vi "ProbeAdjustment.vi"() -> ()   [LabVIEW 2014]
uses:
  <vilib>/rvi/Emulation/niFpgaSctlEmulationGetInTimedLoop.vi
  <vilib>/rvi/Emulation/niFpgaProcessEmulError.vi
  <vilib>/rvi/eio/common/nirviEmuTemplateMethod_errors.vi
  <vilib>/rvi/Emulation/niFpgaGetClockAttributes.vi
  <vilib>/rvi/Emulation/niFpgaEmulationReportErrorSimple.vi
  <vilib>/rvi/Emulation/niFpgaCriticalErrorInLSC.vi
  <vilib>/eio/EIONode/EIONode.xnode
panel:
  out "NewRefCurrIndex":i16
  out "preCurrIndex":i16
  out "Reversing?":bool=TRUE
  in  "Terminal":bool=TRUE
  out "InPlace?":bool
  out "Approached?":bool
  in  "stop":bool
  out "PIZPos":i16
  in  "ProbeBrokenIndex":i16
  in  "ScanNumToRefresh":i16
  in  "ThresholdIndex":i16
  in  "stepMultiplier/0.305nm":i16
  in  "refCurrIndex":i16
  in  "Sleep ms":i16
  in  "ThresholdLowerBound":i16
  in  "ThresholdUpperBound":i16
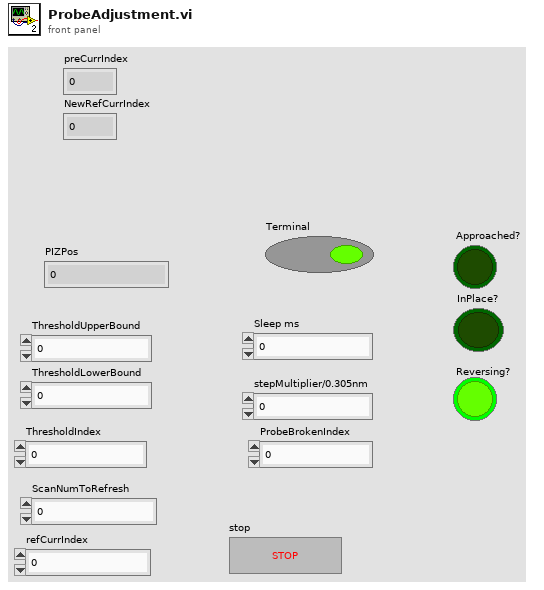
[diagram p1: front panel]
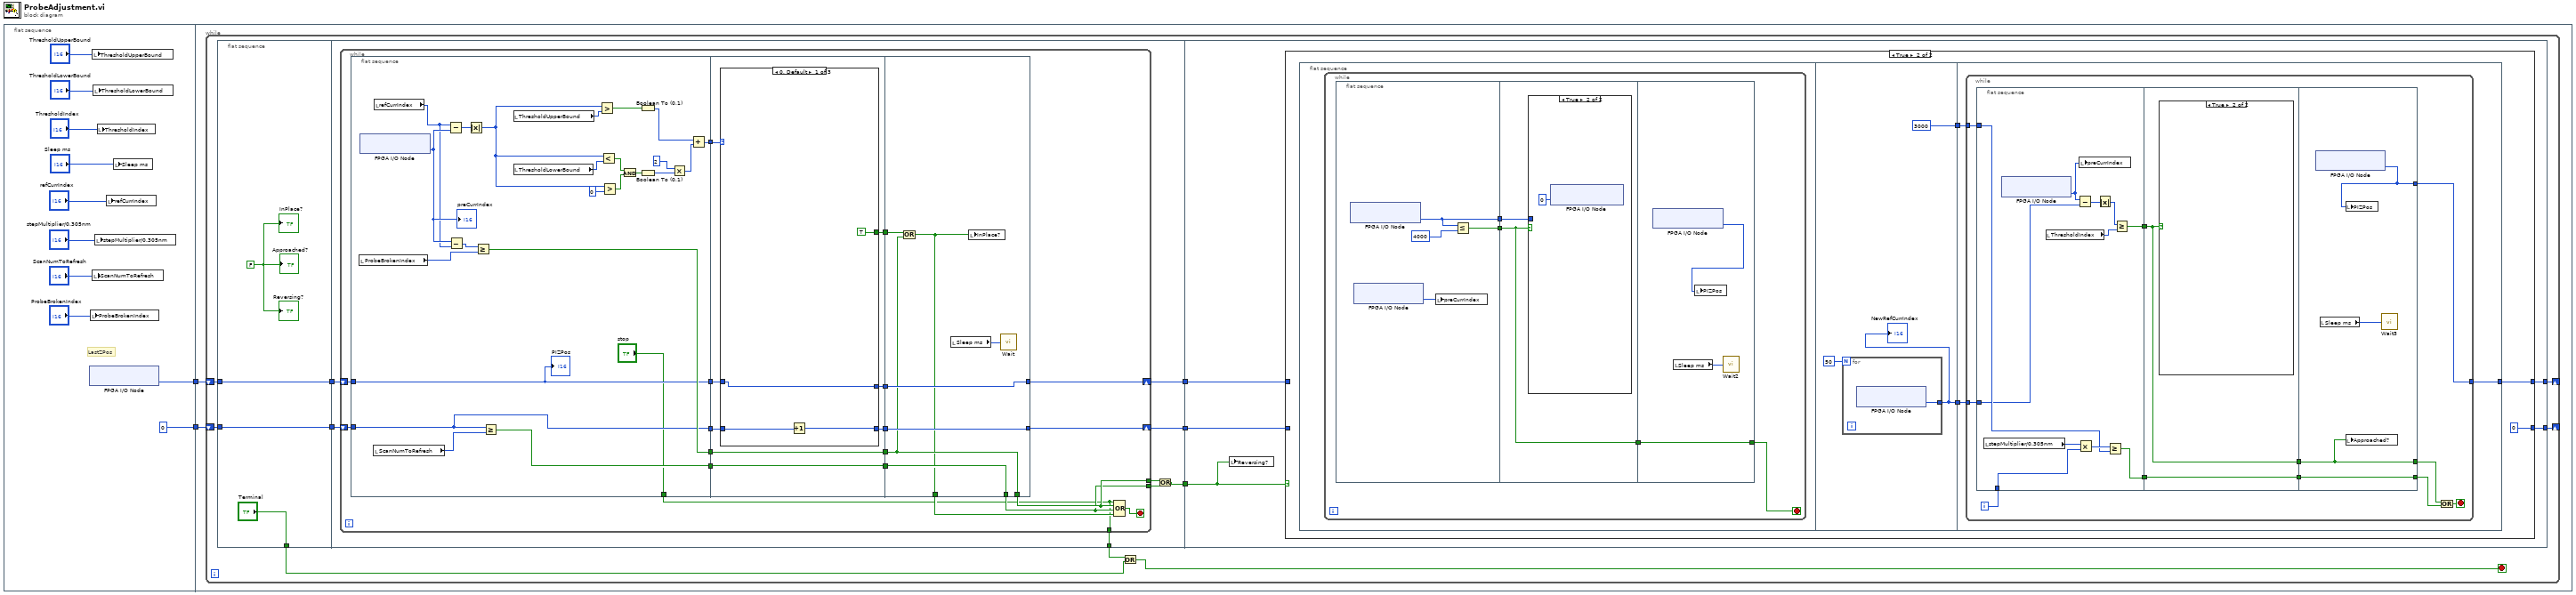
[diagram p0: block diagram]
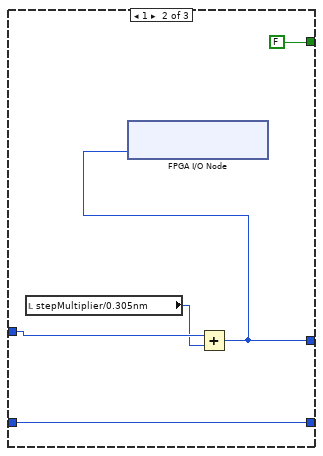
[diagram p2: hidden frame]
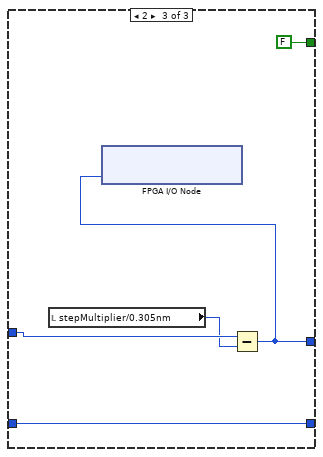
[diagram p3: hidden frame]
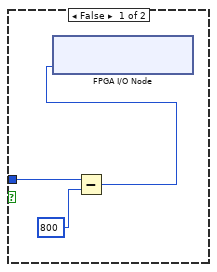
[diagram p5: hidden frame]
diagram:
  n1 = flat-sequence {
    tunnel: [w4] -> w2
    tunnel: [i16 0] -> w1
    tunnel: w2 -> [w13]
    tunnel: w1 -> [w14]
    frame #0 {
      # "LastZPos"
      n2 = xnode "FPGA I/O Node"() -> ("Connector0/AI0"=w4:i16)  [unwired: 1 in, 1 out]
      n3 = local write "ProbeBrokenIndex"("ProbeBrokenIndex") -> ()
      n4 = local write "ThresholdUpperBound"("ThresholdUpperBound") -> ()
      n5 = local write "ScanNumToRefresh"("ScanNumToRefresh") -> ()
      n6 = local write "ThresholdLowerBound"("ThresholdLowerBound") -> ()
      n7 = local write "stepMultiplier/0.305nm"("stepMultiplier/0.305nm") -> ()
      n8 = local write "ThresholdIndex"("ThresholdIndex") -> ()
      n9 = local write "refCurrIndex"("refCurrIndex") -> ()
      n10 = local write "Sleep ms"("Sleep ms") -> ()
    }
    frame #1 {
      n11 = while {
        shift-right: [w22] -> _
        shift-left: w14 -> [w26]
        shift-right: [w20] -> _
        shift-left: w13 -> [w25]
        stop <- w15 stop-if-true
        n12 = flat-sequence {
          tunnel: w25 -> [w29]
          tunnel: w26 -> [w30]
          tunnel: [w30] -> w24
          tunnel: [w29] -> w23
          tunnel: ["Terminal"] -> w16
          tunnel: [w36] -> w17
          tunnel: w24 -> [w38]
          tunnel: w23 -> [w37]
          tunnel: [w35] -> w21
          tunnel: [w34] -> w19
          tunnel: [w31] -> w18
          tunnel: w21 -> [w114]
          tunnel: w19 -> [w112]
          tunnel: [w115] -> w22
          tunnel: [w113] -> w20
          tunnel: w18 -> [w111]
          frame #0 {
            w27 = FALSE
            "Approached?" <- w27
            "InPlace?" <- w27
            "Reversing?" <- w27
          }
          frame #1 {
            n13 = while {
              shift-right: [w46] -> w34
              shift-left: w37 -> [w52]
              shift-right: [w48] -> w35
              shift-left: w38 -> [w53]
              tunnel: [w39] -> w36
              tunnel: [w41] -> w33
              tunnel: [w40] -> w32
              stop <- w43 stop-if-true
              n14 = flat-sequence {
                tunnel: [w66] -> w57
                tunnel: [w63] -> w54
                tunnel: w53 -> [w59]
                tunnel: w52 -> [w62]
                tunnel: [w62] -> w51
                tunnel: [w59] -> w50
                tunnel: [w60] -> w45
                tunnel: ["stop"] -> w39
                tunnel: w57 -> [w89]
                tunnel: [w88] -> w56
                tunnel: [w87] -> w55
                tunnel: w54 -> [w87]
                tunnel: w51 -> [w86]
                tunnel: w50 -> [w83]
                tunnel: [w84] -> w49
                tunnel: [w85] -> w47
                tunnel: w45 -> [w82]
                tunnel: [w82] -> w44
                tunnel: w56 -> [w109]
                tunnel: w55 -> [w106]
                tunnel: w49 -> [w107]
                tunnel: [w107] -> w48
                tunnel: [w108] -> w46
                tunnel: w47 -> [w108]
                tunnel: [w106] -> w41
                tunnel: [w105] -> w40
                tunnel: w44 -> [w105]
                tunnel: [w104] -> w42
                frame #0 {
                  n15 = local read "ProbeBrokenIndex"() -> (w64:i16)
                  n16 = xnode "FPGA I/O Node"() -> ("Connector0/AI1"=w78:i16)  [unwired: 1 in, 1 out]
                  "preCurrIndex" <- w78
                  n17 = local read "ScanNumToRefresh"() -> (w61:i16)
                  n18 = local read "refCurrIndex"() -> (w77:i16)
                  n19 = Subtract(x=w77, y=w78) -> (x-y=w79:i16)
                  n20 = Subtract(x=w78, y=w77) -> (x-y=w65:i16)
                  n21 = Absolute Value(x=w79) -> (abs(x)=w76:i16)
                  n22 = Greater Or Equal?(x=w65, y=w64) -> (x >= y?=w63:bool)
                  n23 = Greater Or Equal?(x=w59, y=w61) -> (x >= y?=w60:bool)
                  n24 = local read "ThresholdUpperBound"() -> (w81:i16)
                  n25 = local read "ThresholdLowerBound"() -> (w80:i16)
                  n26 = Greater?(x=w76, y=w81) -> (0:w69:bool)
                  n27 = Less?(x=w76, y=w80) -> (x < y?=w74:bool)
                  n28 = Greater?(x=w76, y=i16 0) -> (0:w73:bool)
                  n29 = And(x=w74, y=w73) -> (x .and. y?=w72:bool)
                  n30 = Boolean To (0,1)(Boolean=w69) -> (0, 1=w67:i16)
                  n31 = Boolean To (0,1)(Boolean=w72) -> (0, 1=w71:i16)
                  n32 = Multiply(x=i16 2, y=w71) -> (x*y=w68:i16)
                  n33 = Add(x=w67, y=w68) -> (x+y=w66:i16)
                  "PIZPos" <- w62
                }
                frame #1 {
                  n34 = case shown="0, Default" w89 {
                    tunnel: [TRUE FALSE FALSE] -> w88
                    tunnel: w86 -> [w92 w97 w102]
                    tunnel: [w92 w94 w99] -> w85
                    tunnel: [w90 w95 w100] -> w84
                    tunnel: w83 -> [w91 w95 w100]
                    frame 0, Default {
                      n35 = Increment(x=w91) -> (x+1=w90:i16)
                    }
                    frame 1 {
                      n36 = local read "stepMultiplier/0.305nm"() -> (w96:i16)
                      n37 = Add(x=w97, y=w96) -> (x+y=w94:i16)
                      n38 = xnode "FPGA I/O Node"("Connector0/AO0"=w94) -> ()  [unwired: 1 in, 1 out]
                    }
                    frame 2 {
                      n39 = local read "stepMultiplier/0.305nm"() -> (w101:i16)
                      n40 = Subtract(x=w102, y=w101) -> (x-y=w99:i16)
                      n41 = xnode "FPGA I/O Node"("Connector0/AO0"=w99) -> ()  [unwired: 1 in, 1 out]
                    }
                  }
                }
                frame #2 {
                  n42 = Compound Arithmetic op=OR(w109, w106) -> (w104:bool)
                  n43 = local read "Sleep ms"() -> (w110:i16)
                  n44 = local write "InPlace?"(w104) -> ()
                  n45 = call "Wait"("Count(mSec)"=w110) -> ()  [unwired: 1 out]
                }
              }
              n46 = Compound Arithmetic op=OR(w39, w41, w40, w42) -> (w43:bool)
            }
            n47 = Or(x=w33, y=w32) -> (x .or. y?=w31:bool)
          }
          frame #2 {
            n48 = local write "Reversing?"(w111) -> ()
            n49 = case shown="True" w111 {
              tunnel: [w116 i16 0] -> w115
              tunnel: w114 -> [w116 _]
              tunnel: [w117 w118] -> w113
              tunnel: w112 -> [w117 _]
              frame False {
              }
              frame True {
                n50 = flat-sequence {
                  tunnel: [w139] -> w121
                  tunnel: [i16 3000] -> w120
                  tunnel: w121 -> [w145]
                  tunnel: w120 -> [w144]
                  tunnel: [w143] -> w118
                  frame #0 {
                    n51 = while {
                      stop <- w122 stop-if-true
                      n52 = flat-sequence {
                        tunnel: [w128] -> w125
                        tunnel: [w127] -> w124
                        tunnel: w125 -> [w131]
                        tunnel: w124 -> [w130]
                        tunnel: [w130] -> w123
                        tunnel: w123 -> [w136]
                        tunnel: [w136] -> w122
                        frame #0 {
                          n53 = xnode "FPGA I/O Node"() -> ("Connector0/AI0"=w128:i16)  [unwired: 1 in, 1 out]
                          n54 = xnode "FPGA I/O Node"() -> ("Connector0/AI1"=w126:i16)  [unwired: 1 in, 1 out]
                          n55 = local write "preCurrIndex"(w126) -> ()
                          n56 = Less Or Equal?(x=w128, y=i16 4000) -> (x <= y?=w127:bool)
                        }
                        frame #1 {
                          n57 = case shown="True" w130 {
                            tunnel: w131 -> [w132 _]
                            frame False {
                              n58 = Subtract(x=w132, y=i16 800) -> (x-y=w133:i16)
                              n59 = xnode "FPGA I/O Node"("Connector0/AO0"=w133) -> ()  [unwired: 1 in, 1 out]
                            }
                            frame True {
                              n60 = xnode "FPGA I/O Node"("Connector0/AO0"=i16 0) -> ()  [unwired: 1 in, 1 out]
                            }
                          }
                        }
                        frame #2 {
                          n61 = xnode "FPGA I/O Node"() -> ("Connector0/AI0"=w137:i16)  [unwired: 1 in, 1 out]
                          n62 = local read "Sleep ms"() -> (w138:i16)
                          n63 = local write "PIZPos"(w137) -> ()
                          n64 = call "Wait2"("Count(mSec)"=w138) -> ()  [unwired: 1 out]
                        }
                      }
                    }
                  }
                  frame #1 {
                    n65 = for {
                      N: 50 -> [_]
                      tunnel: [w142] -> w139
                      n66 = xnode "FPGA I/O Node"() -> ("Connector0/AI1"=w142:i16)  [unwired: 1 in, 1 out]
                    }
                    "NewRefCurrIndex" <- w139
                  }
                  frame #2 {
                    n67 = while {
                      tunnel: w145 -> [w156]
                      tunnel: w144 -> [w155]
                      tunnel: [w146] -> w143
                      i -> [w154]
                      stop <- w150 stop-if-true
                      n68 = flat-sequence {
                        tunnel: w156 -> [w161]
                        tunnel: w155 -> [w164]
                        tunnel: w154 -> [w166]
                        tunnel: [w163] -> w153
                        tunnel: [w158] -> w152
                        tunnel: w153 -> [w169]
                        tunnel: w152 -> [w168]
                        tunnel: [w169] -> w151
                        tunnel: [w168] -> w148
                        tunnel: [w173] -> w149
                        tunnel: w151 -> [w173]
                        tunnel: w148 -> [w171]
                        tunnel: [w171] -> w147
                        tunnel: [w170] -> w146
                        frame #0 {
                          n69 = local read "stepMultiplier/0.305nm"() -> (w167:i16)
                          n70 = xnode "FPGA I/O Node"() -> ("Connector0/AI1"=w157:i16)  [unwired: 1 in, 1 out]
                          n71 = local read "ThresholdIndex"() -> (w159:i16)
                          n72 = Subtract(x=w157, y=w161) -> (x-y=w162:i16)
                          n73 = Multiply(x=w167, y=w166) -> (x*y=w165:i32)
                          n74 = local write "preCurrIndex"(w157) -> ()
                          n75 = Absolute Value(x=w162) -> (abs(x)=w160:i16)
                          n76 = Greater Or Equal?(x=w165, y=w164) -> (x >= y?=w163:bool)
                          n77 = Greater Or Equal?(x=w160, y=w159) -> (x >= y?=w158:bool)
                        }
                        frame #1 {
                          n78 = case shown="True" w168 {
                            frame False {
                            }
                            frame True {
                            }
                          }
                        }
                        frame #2 {
                          n79 = xnode "FPGA I/O Node"() -> ("Connector0/AI1"=w170:i16)  [unwired: 1 in, 1 out]
                          n80 = local read "Sleep ms"() -> (w172:i16)
                          n81 = local write "PIZPos"(w170) -> ()
                          n82 = local write "Approached?"(w171) -> ()
                          n83 = call "Wait3"("Count(mSec)"=w172) -> ()  [unwired: 1 out]
                        }
                      }
                      n84 = Or(x=w147, y=w149) -> (x .or. y?=w150:bool)
                    }
                  }
                }
              }
            }
          }
        }
        n85 = Or(x=w17, y=w16) -> (x .or. y?=w15:bool)
      }
    }
  }
